vi "requestStop.vi"(8 "error in (no error)":errorcluster, 11 "NotifierStopMechanism in":refnum<class "BoolNotifierTaskChannel.lvclass">) -> (0 "error out":errorcluster, 3 "NotifierStopMechanism out":refnum<class "BoolNotifierTaskChannel.lvclass">)   [LabVIEW 2023, in "TLC_Daemon.lvlib" / "BoolNotifierTaskChannel.lvclass"]
doc: "Triggers a stop request for a target task."
uses:
  BoolNotifierTaskChannel.lvclass
  BoolNotifierTaskChannel.lvclass/BoolNotifierTaskChannel.ctl
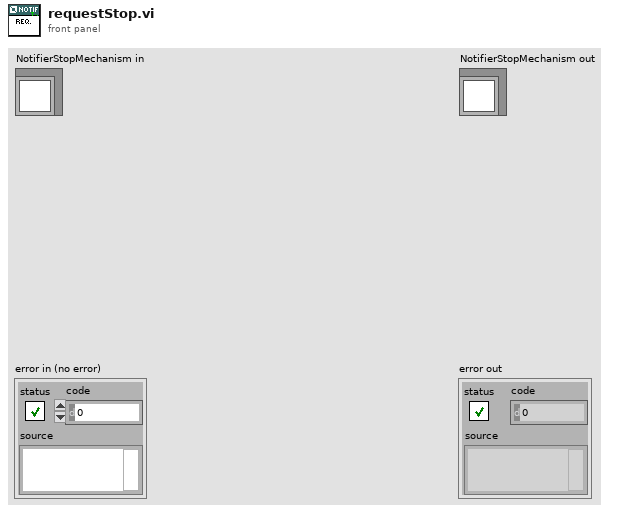
[diagram p1: front panel]
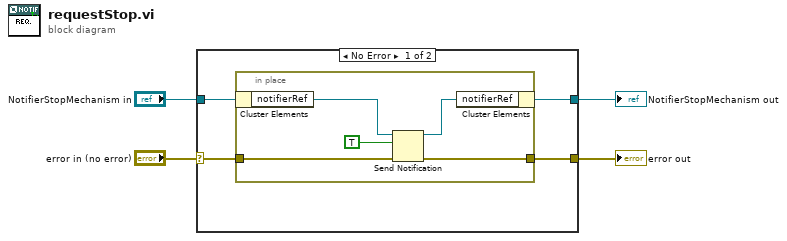
[diagram p0: block diagram]
diagram:
  n1 = case shown="No Error" "error in (no error)" {
    selector: "error in (no error)" -> [w7 w15]
    tunnel: [w6 w15] -> w3
    tunnel: "NotifierStopMechanism in" -> [w8 w14]
    tunnel: [w5 w14] -> w1
    frame No Error {
      n2 = in-place {
        in-place-border: w7 -> [w10]
        in-place-border: [w9] -> w6
        n3 = in-place-cluster #1(w8) -> ("notifierRef"=w13:refnum<notifier>)
        n4 = Send Notification(notification=TRUE, notifier=w13, error in (no error)=w10) -> (notifier out=w12:refnum<notifier>, error out=w9:errorcluster)
        n5 = in-place-cluster #1("notifierRef"=w12) -> (w5:refnum<class "BoolNotifierTaskChannel.lvclass">)
      }
    }
    frame Error {
    }
  }
  "error out" <- w3
  "NotifierStopMechanism out" <- w1
